vi "Send Robot State.vi"(11 "CurrentState":T1(ring)) -> ()   [LabVIEW 2013]
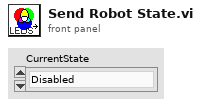
[diagram p1: front panel]
types:
  T1 = enum16{"Disabled", "Teleop", "Spinning Wheels", "Moving Arm", "Shooting", "Success"}
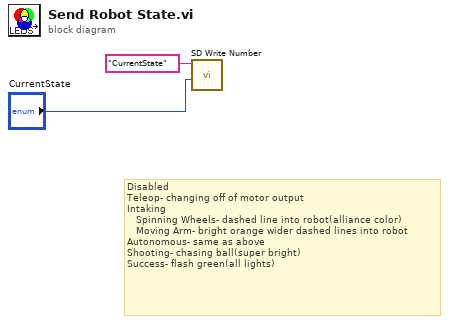
[diagram p0: block diagram]
diagram:
  # "Disabled\nTeleop- changing off of motor output\nIntaking\n\t  Spinning Wheels- dashed line into robot(alliance color)\n\t  Moving Arm- bright orange wider dashed lines into robot\nAutonomous- same as above\nShooting- chasing ball(super bright)\nSuccess- flash green(all lights)"
  n1 = call <vilib>:"SD Write Number.vi"("Numeric"="CurrentState", "Name"="CurrentState") -> ()  [unwired: 8 in, 2 out]
